vi "RTS Build Door Ops Path.vi"(8 "Error In":errorcluster, 10 "System Number":T1="Select System", 11 "Search File Path Input":path) -> (0 "Error Out":errorcluster, 3 "appended path":path)   [LabVIEW 2016]
uses:
  Type Definitions/RTS Select System Number.ctl
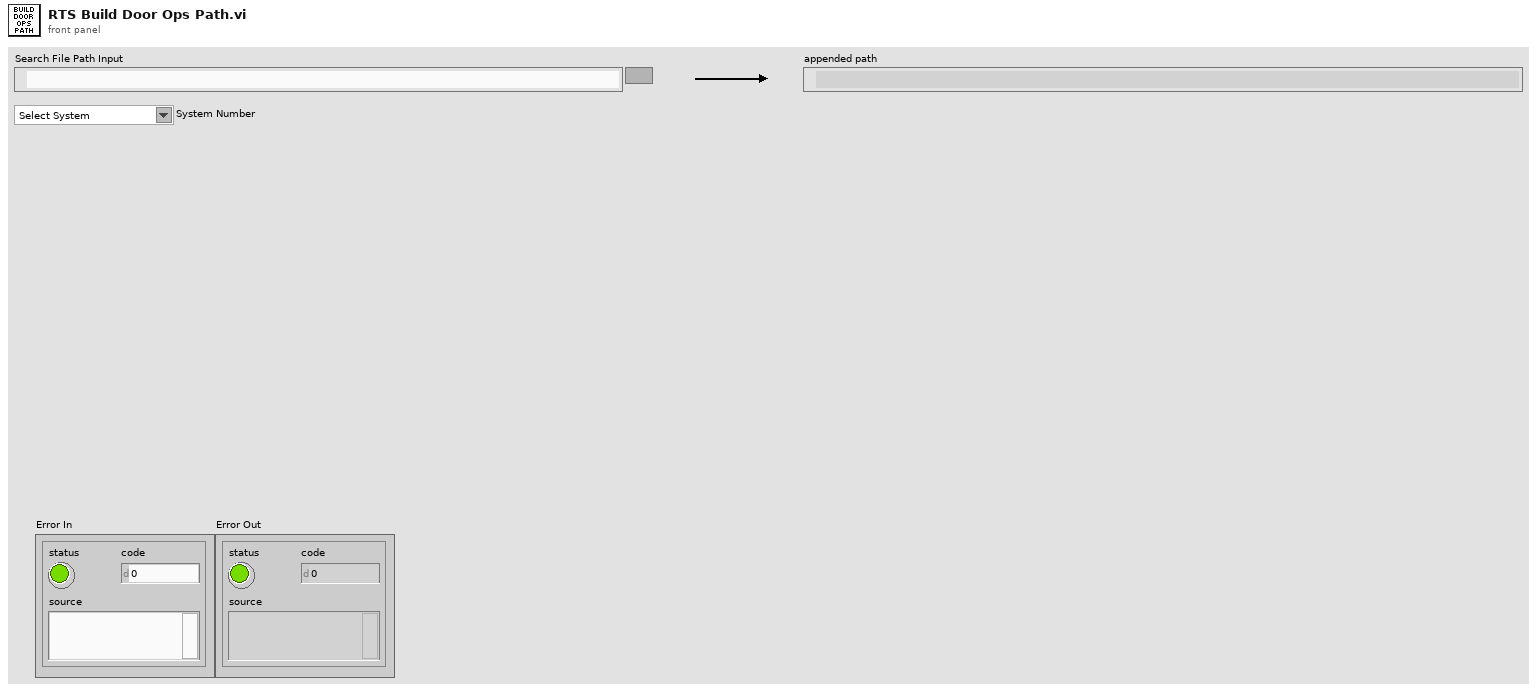
[diagram p1: front panel]
types:
  T1 = typedef "RTS Select System Number.ctl" = string
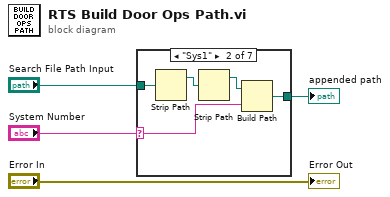
[diagram p0: block diagram]
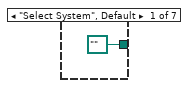
[diagram p2: hidden frame]
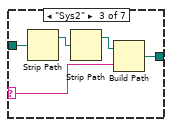
[diagram p3: hidden frame]
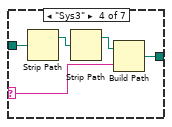
[diagram p4: hidden frame]
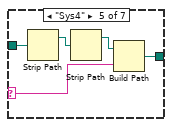
[diagram p5: hidden frame]
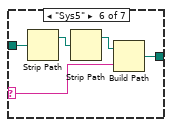
[diagram p6: hidden frame]
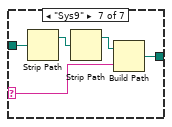
[diagram p7: hidden frame]
diagram:
  n1 = case shown="\"Sys1\"" "System Number" {
    selector: "System Number" -> [_ w7 w12 w17 w22 w27 w32]
    tunnel: "Search File Path Input" -> [_ w8 w13 w18 w23 w28 w35]
    tunnel: [path "" ("appended path") w6 w11 w16 w21 w26 w31] -> w4
    frame "Select System", Default {
    }
    frame "Sys1" {
      n2 = Strip Path(path=w8) -> (stripped path=w10:path)  [unwired: 1 out]
      n3 = Strip Path(path=w10) -> (stripped path=w9:path)  [unwired: 1 out]
      n4 = Build Path(base path=w9, name or relative path=w7) -> (appended path=w6:path)
    }
    frame "Sys2" {
      n5 = Strip Path(path=w13) -> (stripped path=w15:path)  [unwired: 1 out]
      n6 = Strip Path(path=w15) -> (stripped path=w14:path)  [unwired: 1 out]
      n7 = Build Path(base path=w14, name or relative path=w12) -> (appended path=w11:path)
    }
    frame "Sys3" {
      n8 = Strip Path(path=w18) -> (stripped path=w20:path)  [unwired: 1 out]
      n9 = Strip Path(path=w20) -> (stripped path=w19:path)  [unwired: 1 out]
      n10 = Build Path(base path=w19, name or relative path=w17) -> (appended path=w16:path)
    }
    frame "Sys4" {
      n11 = Strip Path(path=w23) -> (stripped path=w25:path)  [unwired: 1 out]
      n12 = Strip Path(path=w25) -> (stripped path=w24:path)  [unwired: 1 out]
      n13 = Build Path(base path=w24, name or relative path=w22) -> (appended path=w21:path)
    }
    frame "Sys5" {
      n14 = Strip Path(path=w28) -> (stripped path=w30:path)  [unwired: 1 out]
      n15 = Strip Path(path=w30) -> (stripped path=w29:path)  [unwired: 1 out]
      n16 = Build Path(base path=w29, name or relative path=w27) -> (appended path=w26:path)
    }
    frame "Sys9" {
      n17 = Strip Path(path=w35) -> (stripped path=w34:path)  [unwired: 1 out]
      n18 = Strip Path(path=w34) -> (stripped path=w33:path)  [unwired: 1 out]
      n19 = Build Path(base path=w33, name or relative path=w32) -> (appended path=w31:path)
    }
  }
  "appended path" <- w4
  "Error Out" <- "Error In"
